vi "LPC Main 1.0.vi"() -> ()   [LabVIEW 2009]
doc: "Main control panel for the laser power controller."
uses:
  BEOC LPC/BEOC LPC.lvlib
panel:
  in  "Set front-panel controls":bool
  in  "Set Wavelength":bool
  in  "Set Transmission":bool
  in  "Set Control Mode":bool
  in  "Set Power":bool
  out "?":dbl
  in  "Transmission":dbl=50.0
  in  "read":bool
  out "front-panel controls":enum16{"enabled", "disabled"}(ring)
  in  "front-panel controls":enum16{"enabled", "disabled"}(ring)
  out "control mode":T1(ring)
  in  "control mode":T1(ring)
  out "wavelength":dbl[unit]
  in  "wavelength":dbl[unit]=8.300000000000001e-07
  out "power":dbl[unit]
  in  "power":dbl[unit]=0.005
  in  "exit":bool
  out "Online":bool caption="online"
  out "Reading":bool
  # "Laser Power Controller (LPC)"
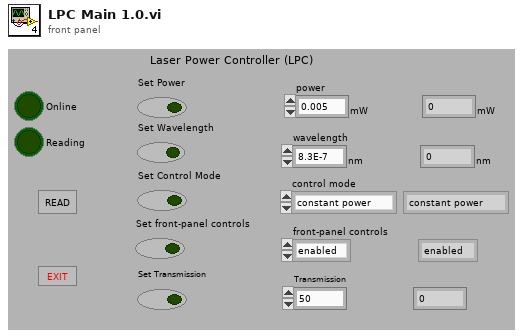
[diagram p1: front panel]
types:
  T1 = enum16{"constant power", "constant transmission"}
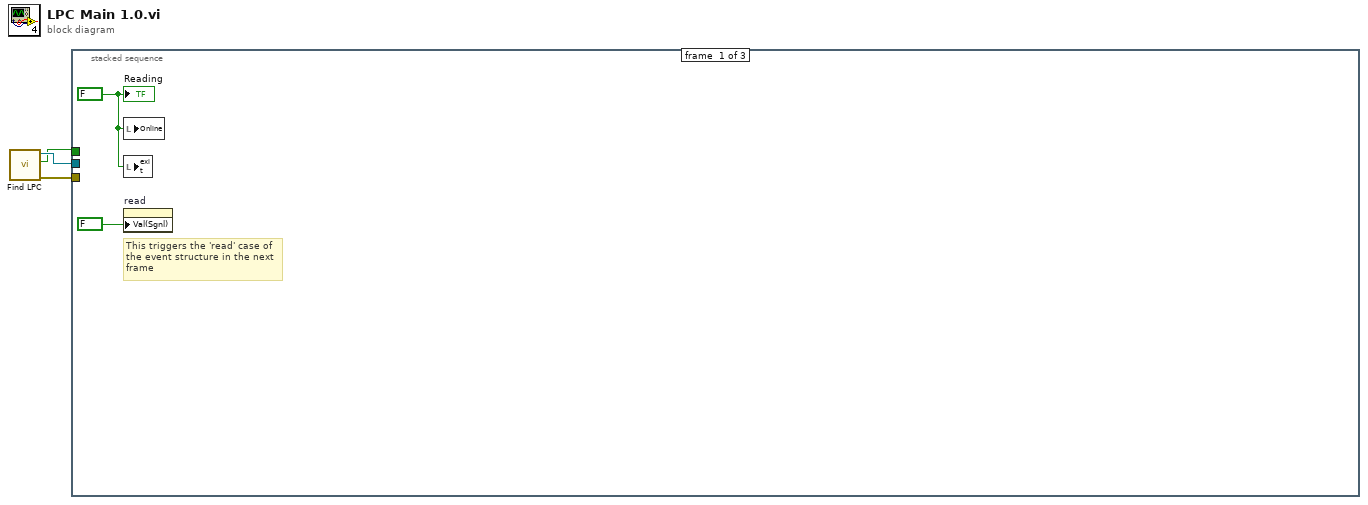
[diagram p0: block diagram]
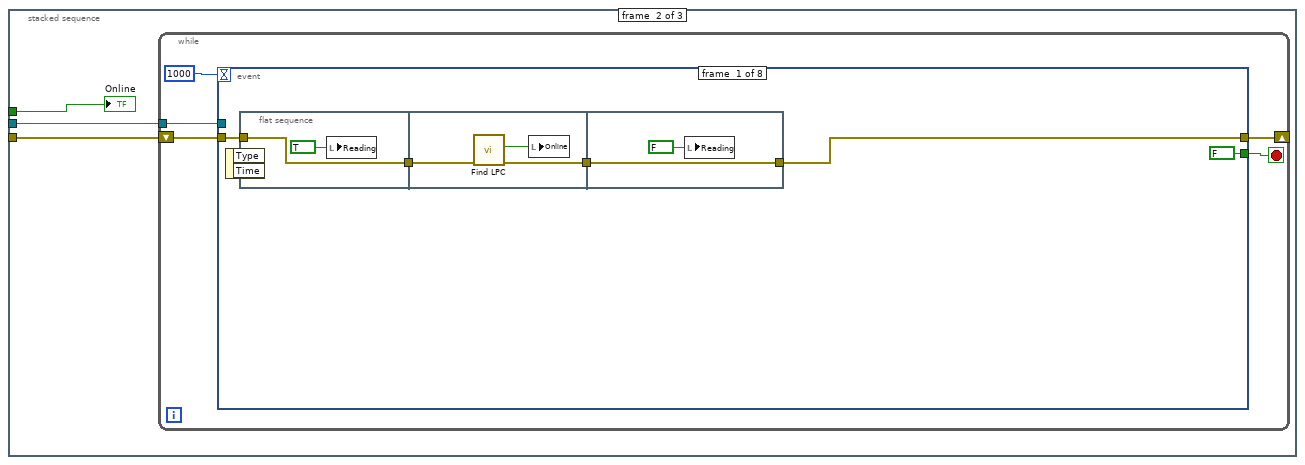
[diagram p2: hidden frame]
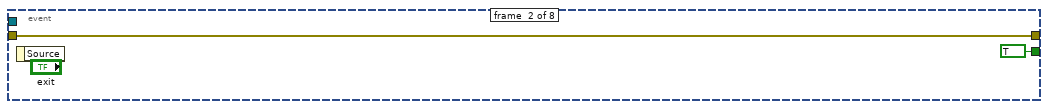
[diagram p3: hidden frame]
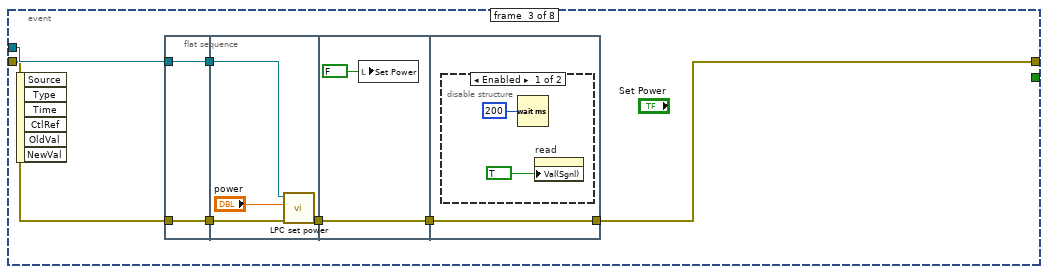
[diagram p4: hidden frame]
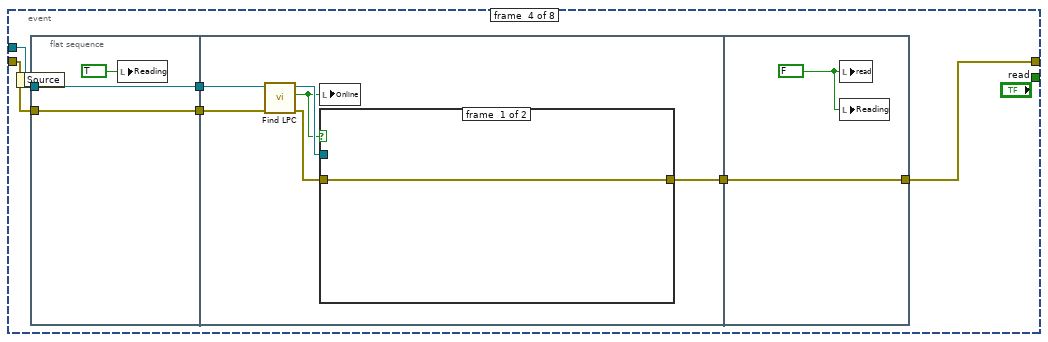
[diagram p6: hidden frame]
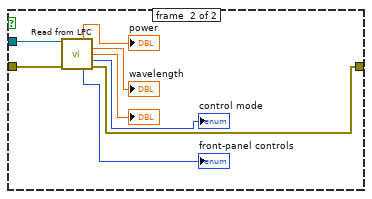
[diagram p7: hidden frame]
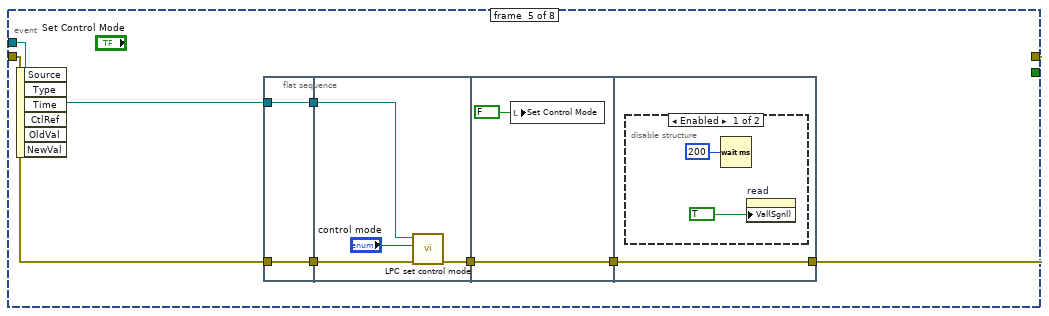
[diagram p8: hidden frame]
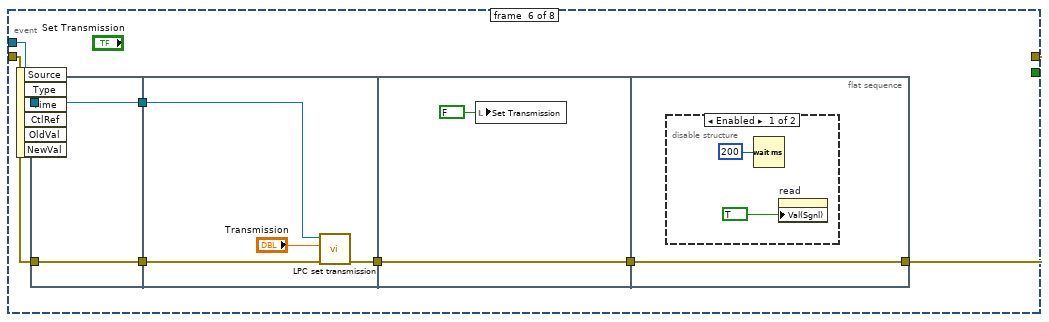
[diagram p10: hidden frame]
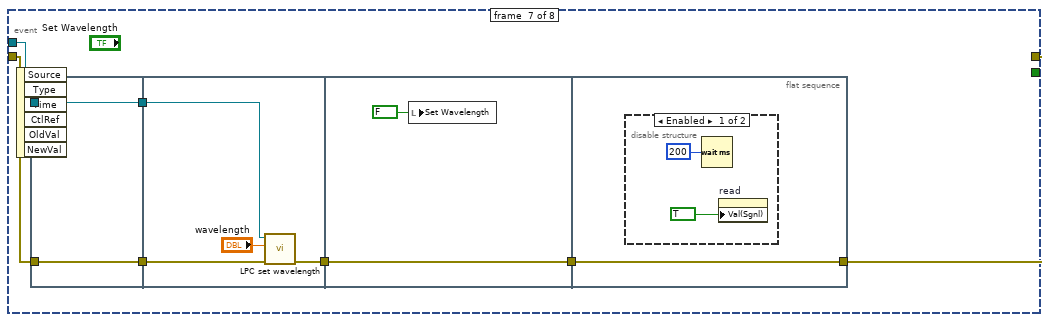
[diagram p12: hidden frame]
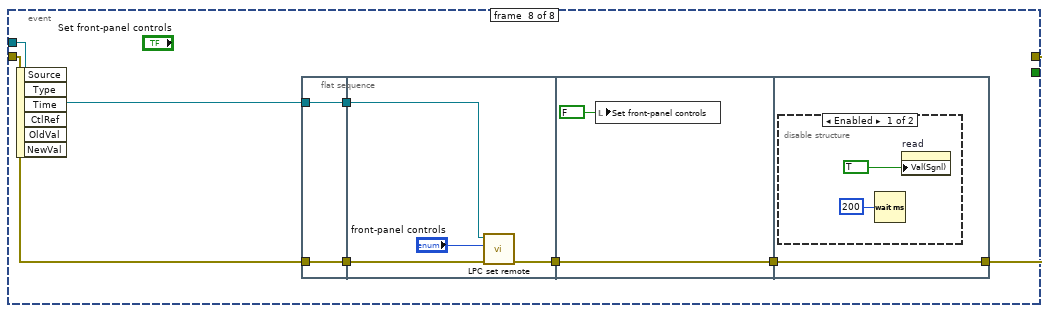
[diagram p14: hidden frame]
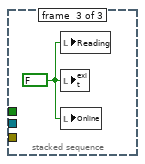
[diagram p16: hidden frame]
diagram:
  n1 = call "Find LPC.vi"() -> ("error out"=w1:errorcluster, "LPC found?"=w2:bool, "VISA resource name out"=w3:refnum<visa-resource-name>)  [unwired: 2 in, 7 out]
  n2 = stacked-sequence {
    tunnel: w3 -> [_ w6 _]
    tunnel: w2 -> [_ w8 _]
    tunnel: w1 -> [_ w7 _]
    frame #0 {
      w5 = FALSE ("Reading")
      # "This triggers the 'read' case of the event structure in the next frame"
      n3 = local write "Online"(w5) -> ()
      n4 = local write "exit"(w5) -> ()
      n5 = property on="read" class="Bool (strict)"("Val(Sgnl)"=FALSE ("Value (Signaling)")) -> ()  [unwired: 2 in, 2 out]
      "Reading" <- w5
    }
    frame #1 {
      n6 = while {
        shift-right: [w11] -> _
        shift-left: w7 -> [w12]
        tunnel: w6 -> [w9]
        stop <- w10 stop-if-true
        n7 = event shown="[2] \"Set Power\": Value Change" {
          selector: _ -> [_ _ _ _ _ _ _ _]
          dyn-events: _ -> [_ _ _ _ _ _ _ _]
          timeout: 1000 -> [_ _ _ _ _ _ _ _]
          tunnel: w12 -> [w18 w26 w33 w50 w78 w95 w113 w131]
          tunnel: [w17 w26 w32 w46 w77 w94 w112 w130] -> w11
          tunnel: [FALSE TRUE _ _ _ _ _ _] -> w10
          tunnel: w9 -> [_ _ w34 w51 w76 w96 w114 w132]
          event #0 {
            n8 = event-data() -> ()  [unwired: 3 out]
            n9 = flat-sequence {
              tunnel: w18 -> [w20]
              tunnel: [w20] -> w15
              tunnel: w15 -> [w23]
              tunnel: [w21] -> w14
              tunnel: [w25] -> w17
              tunnel: w14 -> [w25]
              frame #0 {
                n10 = local write "Reading"(TRUE ("Reading")) -> ()
              }
              frame #1 {
                n11 = call "Find LPC.vi"("error in (no error)"=w23) -> ("error out"=w21:errorcluster, "LPC found?"=w22:bool)  [unwired: 1 in, 8 out]
                n12 = local write "Online"(w22) -> ()
              }
              frame #2 {
                n13 = local write "Reading"(FALSE ("Reading")) -> ()
              }
            }
          }
          event #1 {
            n14 = event-data() -> ()  [unwired: 2 out]
          }
          event #2 {
            n15 = event-data() -> ()  [unwired: 7 out]
            n16 = flat-sequence {
              tunnel: w33 -> [w35]
              tunnel: w34 -> [w36]
              tunnel: [w36] -> w31
              tunnel: [w35] -> w30
              tunnel: w31 -> [w40]
              tunnel: w30 -> [w39]
              tunnel: [w38] -> w29
              tunnel: w29 -> [w42]
              tunnel: [w42] -> w28
              tunnel: [w43] -> w32
              tunnel: w28 -> [w43]
              frame #0 {
              }
              frame #1 {
                n17 = call "LPC set power.vi"("error in (no error)"=w39, "power"="power", "VISA resource name"=w40) -> ("error out"=w38:errorcluster)  [unwired: 7 in, 1 out]
              }
              frame #2 {
                n18 = local write "Set Power"(FALSE ("Set Power")) -> ()
              }
              frame #3 {
                n19 = disable-structure shown="Enabled" {
                  frame #0 {
                    n20 = Wait (ms)(milliseconds to wait=u32 200) -> ()  [unwired: 1 out]
                    n21 = property on="read" class="Bool (strict)"("Val(Sgnl)"=TRUE ("Value (Signaling)")) -> ()  [unwired: 2 in, 2 out]
                  }
                  frame #1 {
                  }
                }
              }
            }
          }
          event #3 {
            n22 = event-data() -> ()  [unwired: 2 out]
            n23 = flat-sequence {
              tunnel: w50 -> [w53]
              tunnel: w51 -> [w54]
              tunnel: [w54] -> w49
              tunnel: [w53] -> w48
              tunnel: w49 -> [w56]
              tunnel: w48 -> [w59]
              tunnel: [w60] -> w47
              tunnel: w47 -> [w71]
              tunnel: [w71] -> w46
              frame #0 {
                n24 = local write "Reading"(TRUE ("Reading")) -> ()
              }
              frame #1 {
                n25 = call "Find LPC.vi"("error in (no error)"=w59, "VISA resource name"=w56) -> ("error out"=w58:errorcluster, "LPC found?"=w55:bool, "VISA resource name out"=w57:refnum<visa-resource-name>)  [unwired: 7 out]
                n26 = local write "Online"(w55) -> ()
                n27 = case shown="True" w55 {
                  tunnel: [w61 w69] -> w60
                  tunnel: w58 -> [w61 w64]
                  tunnel: w57 -> [_ w63]
                  frame #0 {
                  }
                  frame #1 {
                    n28 = call "Read from LPC.vi"("VISA resource name"=w63, "error in (no error)"=w64) -> ("power"=→"power":dbl[unit], "wavelength"=→"wavelength":dbl[unit], "Transmission"=→"?":dbl, "control mode"=→"control mode":T1, "front-panel controls"=→"front-panel controls":enum16{"enabled", "disabled"}, "error out"=w69:errorcluster)  [unwired: 7 in, 1 out]
                  }
                }
              }
              frame #2 {
                w70 = FALSE ("Reading")
                n29 = local write "read"(w70) -> ()
                n30 = local write "Reading"(w70) -> ()
              }
            }
          }
          event #4 {
            n31 = event-data() -> ()  [unwired: 7 out]
            n32 = flat-sequence {
              tunnel: w76 -> [w79]
              tunnel: w78 -> [w80]
              tunnel: [w80] -> w73
              tunnel: [w79] -> w72
              tunnel: [w83] -> w75
              tunnel: w73 -> [w84]
              tunnel: w72 -> [w82]
              tunnel: w75 -> [w86]
              tunnel: [w86] -> w74
              tunnel: [w87] -> w77
              tunnel: w74 -> [w87]
              frame #0 {
              }
              frame #1 {
                n33 = call "LPC set control mode.vi"("error in (no error)"=w84, "control mode"="control mode", "VISA resource name"=w82) -> ("error out"=w83:errorcluster)  [unwired: 7 in, 1 out]
              }
              frame #2 {
                n34 = local write "Set Control Mode"(FALSE ("Set Control Mode")) -> ()
              }
              frame #3 {
                n35 = disable-structure shown="Enabled" {
                  frame #0 {
                    n36 = Wait (ms)(milliseconds to wait=u32 200) -> ()  [unwired: 1 out]
                    n37 = property on="read" class="Bool (strict)"("Val(Sgnl)"=TRUE ("Value (Signaling)")) -> ()  [unwired: 2 in, 2 out]
                  }
                  frame #1 {
                  }
                }
              }
            }
          }
          event #5 {
            n38 = event-data() -> ()  [unwired: 7 out]
            n39 = flat-sequence {
              tunnel: w95 -> [w97]
              tunnel: w96 -> [w98]
              tunnel: [w98] -> w91
              tunnel: [w97] -> w90
              tunnel: [w100] -> w93
              tunnel: w91 -> [w102]
              tunnel: w90 -> [w101]
              tunnel: w93 -> [w104]
              tunnel: [w104] -> w92
              tunnel: [w105] -> w94
              tunnel: w92 -> [w105]
              frame #0 {
              }
              frame #1 {
                n40 = call "LPC set transmission.vi"("error in (no error)"=w101, "transmission (%)"="Transmission", "VISA resource name"=w102) -> ("error out"=w100:errorcluster)  [unwired: 7 in, 1 out]
              }
              frame #2 {
                n41 = local write "Set Transmission"(FALSE ("Set Transmission")) -> ()
              }
              frame #3 {
                n42 = disable-structure shown="Enabled" {
                  frame #0 {
                    n43 = Wait (ms)(milliseconds to wait=u32 200) -> ()  [unwired: 1 out]
                    n44 = property on="read" class="Bool (strict)"("Val(Sgnl)"=TRUE ("Value (Signaling)")) -> ()  [unwired: 2 in, 2 out]
                  }
                  frame #1 {
                  }
                }
              }
            }
          }
          event #6 {
            n45 = event-data() -> ()  [unwired: 7 out]
            n46 = flat-sequence {
              tunnel: w113 -> [w115]
              tunnel: w114 -> [w116]
              tunnel: [w116] -> w109
              tunnel: [w115] -> w108
              tunnel: [w118] -> w111
              tunnel: w109 -> [w120]
              tunnel: w108 -> [w119]
              tunnel: w111 -> [w122]
              tunnel: [w122] -> w110
              tunnel: [w123] -> w112
              tunnel: w110 -> [w123]
              frame #0 {
              }
              frame #1 {
                n47 = call "LPC set wavelength.vi"("error in (no error)"=w119, "wavelength"="wavelength", "VISA resource name"=w120) -> ("error out"=w118:errorcluster)  [unwired: 7 in, 1 out]
              }
              frame #2 {
                n48 = local write "Set Wavelength"(FALSE ("Set Wavelength")) -> ()
              }
              frame #3 {
                n49 = disable-structure shown="Enabled" {
                  frame #0 {
                    n50 = Wait (ms)(milliseconds to wait=u32 200) -> ()  [unwired: 1 out]
                    n51 = property on="read" class="Bool (strict)"("Val(Sgnl)"=TRUE ("Value (Signaling)")) -> ()  [unwired: 2 in, 2 out]
                  }
                  frame #1 {
                  }
                }
              }
            }
          }
          event #7 {
            n52 = event-data() -> ()  [unwired: 7 out]
            n53 = flat-sequence {
              tunnel: w131 -> [w133]
              tunnel: w132 -> [w134]
              tunnel: [w134] -> w127
              tunnel: [w133] -> w126
              tunnel: [w136] -> w129
              tunnel: w127 -> [w138]
              tunnel: w126 -> [w137]
              tunnel: w129 -> [w140]
              tunnel: [w140] -> w128
              tunnel: [w141] -> w130
              tunnel: w128 -> [w141]
              frame #0 {
              }
              frame #1 {
                n54 = call "LPC set remote.vi"("error in (no error)"=w137, "front-panel controls"="front-panel controls", "VISA resource name"=w138) -> ("error out"=w136:errorcluster)  [unwired: 7 in, 1 out]
              }
              frame #2 {
                n55 = local write "Set front-panel controls"(FALSE ("Set front-panel controls")) -> ()
              }
              frame #3 {
                n56 = disable-structure shown="Enabled" {
                  frame #0 {
                    n57 = Wait (ms)(milliseconds to wait=u32 200) -> ()  [unwired: 1 out]
                    n58 = property on="read" class="Bool (strict)"("Val(Sgnl)"=TRUE ("Value (Signaling)")) -> ()  [unwired: 2 in, 2 out]
                  }
                  frame #1 {
                  }
                }
              }
            }
          }
        }
      }
      "Online" <- w8
    }
    frame #2 {
      w144 = FALSE ("Reading")
      n59 = local write "Reading"(w144) -> ()
      n60 = local write "exit"(w144) -> ()
      n61 = local write "Online"(w144) -> ()
    }
  }
